vi "item select write disabled.vi"(8 "error in (no error)":errorcluster, 10 "Disabled?":bool[](array[boolean]), 11 "Listbox or Tree":refnum<vi>) -> (0 "error out":errorcluster, 3 "Ref":refnum<vi>)   [LabVIEW 2020, in "UI_ItemSelect_OpenSource.lvlib"]
doc: "This method allows the user to manually write Disabled states.\n\nArray length of Selection must match the array length of:\n<B>Listbox</B>: ItemNames\n<B>MCL</B>: ItemNames column length\n<B>Tree</B>: number of child-only tags"
uses:
  UI_ItemSelect_OpenSource.lvlib
  SubVIs/item select action.ctl
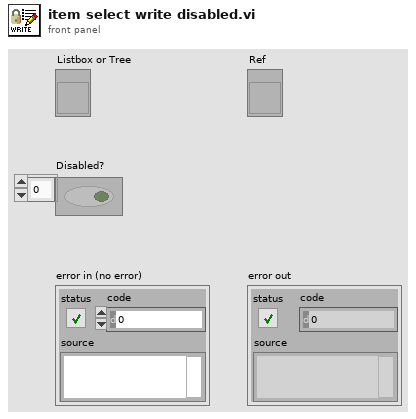
[diagram p1: front panel]
types:
  T1 = typedef "UI_ItemSelect_OpenSource.lvlib/item select action.ctl" = enum16{"init", "read", "write states", "write locks", "mouse down", "delete", "select all", "select none", "invert selection"}
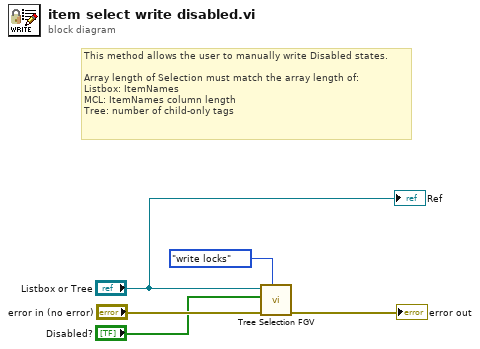
[diagram p0: block diagram]
diagram:
  # "This method allows the user to manually write Disabled states.\n\nArray length of Selection must match the array length of:\nListbox: ItemNames\nMCL: ItemNames column length\nTree: number of child-only tags"
  n1 = call "Tree Selection FGV.vi"("Action"=item_select_action."write locks", "error in (no error)"="error in (no error)", "States"="Disabled?", "Listbox or Tree"="Listbox or Tree") -> ("error out"=→"error out":errorcluster)  [unwired: 6 in, 1 out]
  "Ref" <- "Listbox or Tree"
